vi "scaledImageUINT8.vi"(11 "double image":dbl[][](array[numeric])) -> (3 "uint8 image":u8[][](array[numeric]))   [LabVIEW 2016]
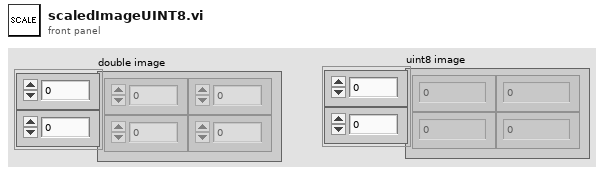
[diagram p1: front panel]
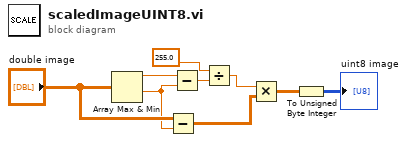
[diagram p0: block diagram]
diagram:
  n1 = Array Max & Min(array="double image") -> (max value=w9:dbl, min value=w5:dbl)  [unwired: 2 out]
  n2 = Subtract(x="double image", y=w5) -> (x-y=w3:dbl[][])
  n3 = Subtract(x=w9, y=w5) -> (x-y=w8:dbl)
  n4 = Divide(x=255.0, y=w8) -> (x/y=w4:dbl)
  n5 = Multiply(x=w4, y=w3) -> (x*y=w2:dbl[][])
  n6 = To Unsigned Byte Integer(number=w2) -> (unsigned 8bit integer=→"uint8 image":u8[][])
